vi "LUT_selector.vi"(2 "LUT 2":T1(ring)=enum."cold/hot (1/2)", 3 "LUT1":T1(ring)=enum."cold/hot (1/2)") -> (0 "Palette 2":cluster{u8, u8, u8}[](array[cluster]), 1 "Palette1":cluster{u8, u8, u8}[](array[cluster]))   [LabVIEW 2013]
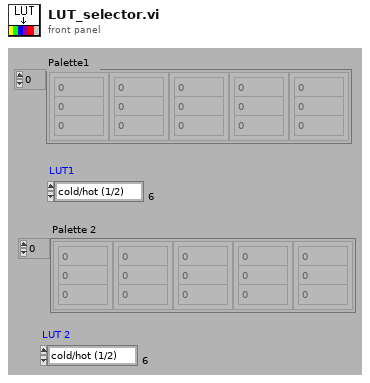
[diagram p1: front panel]
types:
  T1 = enum16{"grey-progress", "gray", "gray + high", "gray + bounds", "gradient", "temperature", "cold/hot (1/2)", "cold/hot (1/4)", "odd/even"}
  T2 = enum32{"Gray", "Binary", "Gradient", "Rainbow", "Temperature"}
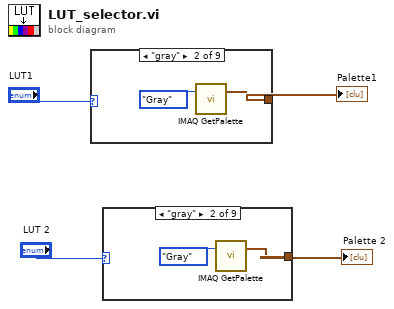
[diagram p0: block diagram]
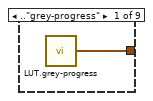
[diagram p2: hidden frame]
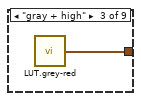
[diagram p3: hidden frame]
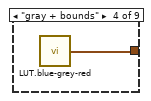
[diagram p4: hidden frame]
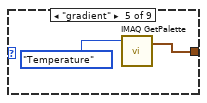
[diagram p5: hidden frame]
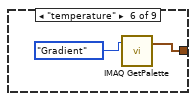
[diagram p6: hidden frame]
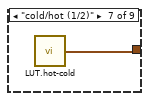
[diagram p7: hidden frame]
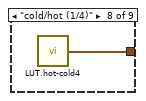
[diagram p8: hidden frame]
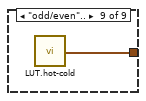
[diagram p9: hidden frame]
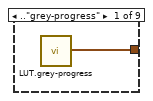
[diagram p10: hidden frame]
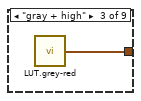
[diagram p11: hidden frame]
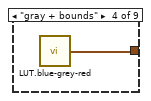
[diagram p12: hidden frame]
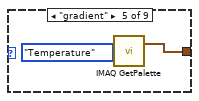
[diagram p13: hidden frame]
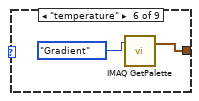
[diagram p14: hidden frame]
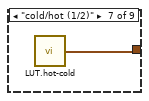
[diagram p15: hidden frame]
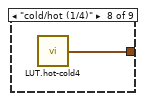
[diagram p16: hidden frame]
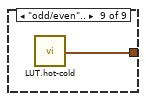
[diagram p17: hidden frame]
diagram:
  n1 = case shown="\"gray\"" "LUT1" {
    tunnel: [w5 w6 w8 w9 w10 w12 w14 w15 w16] -> w4
    frame .."grey-progress" {
      n2 = call "LUT.grey-progress.vi"() -> ("grey-progress"=w5:cluster{u8, u8, u8}[])
    }
    frame "gray" {
      n3 = call "IMAQ GetPalette"("Palette Number (gray)"=T2."Gray") -> ("Color Palette"=w6:cluster{"Red":u8, "Green":u8, "Blue":u8}[])  [unwired: 1 in, 4 out]
    }
    frame "gray + high" {
      n4 = call "LUT.grey-red.vi"() -> ("grey-red Palette"=w8:cluster{u8, u8, u8}[])
    }
    frame "gray + bounds" {
      n5 = call "LUT.blue-grey-red.vi"() -> ("Blue-grey-red Palette"=w9:cluster{u8, u8, u8}[])
    }
    frame "gradient" {
      n6 = call "IMAQ GetPalette"("Palette Number (gray)"=T2."Temperature") -> ("Color Palette"=w10:cluster{"Red":u8, "Green":u8, "Blue":u8}[])  [unwired: 1 in, 4 out]
    }
    frame "temperature" {
      n7 = call "IMAQ GetPalette"("Palette Number (gray)"=T2."Gradient") -> ("Color Palette"=w12:cluster{"Red":u8, "Green":u8, "Blue":u8}[])  [unwired: 1 in, 4 out]
    }
    frame "cold/hot (1/2)" {
      n8 = call "LUT.hot-cold.vi"() -> ("Palette"=w14:cluster{u8, u8, u8}[])
    }
    frame "cold/hot (1/4)" {
      n9 = call "LUT.hot-cold4.vi"() -> ("Palette"=w15:cluster{u8, u8, u8}[])
    }
    frame "odd/even".. {
      n10 = call "LUT.hot-cold.vi"() -> ("Palette"=w16:cluster{u8, u8, u8}[])
    }
  }
  "Palette1" <- w4
  n11 = case shown="\"gray\"" "LUT 2" {
    tunnel: [w17 w18 w20 w21 w23 w24 w26 w27 w28] -> w3
    frame .."grey-progress" {
      n12 = call "LUT.grey-progress.vi"() -> ("grey-progress"=w17:cluster{u8, u8, u8}[])
    }
    frame "gray" {
      n13 = call "IMAQ GetPalette"("Palette Number (gray)"=T2."Gray") -> ("Color Palette"=w18:cluster{"Red":u8, "Green":u8, "Blue":u8}[])  [unwired: 1 in, 4 out]
    }
    frame "gray + high" {
      n14 = call "LUT.grey-red.vi"() -> ("grey-red Palette"=w20:cluster{u8, u8, u8}[])
    }
    frame "gray + bounds" {
      n15 = call "LUT.blue-grey-red.vi"() -> ("Blue-grey-red Palette"=w21:cluster{u8, u8, u8}[])
    }
    frame "gradient" {
      n16 = call "IMAQ GetPalette"("Palette Number (gray)"=T2."Temperature") -> ("Color Palette"=w23:cluster{"Red":u8, "Green":u8, "Blue":u8}[])  [unwired: 1 in, 4 out]
    }
    frame "temperature" {
      n17 = call "IMAQ GetPalette"("Palette Number (gray)"=T2."Gradient") -> ("Color Palette"=w24:cluster{"Red":u8, "Green":u8, "Blue":u8}[])  [unwired: 1 in, 4 out]
    }
    frame "cold/hot (1/2)" {
      n18 = call "LUT.hot-cold.vi"() -> ("Palette"=w26:cluster{u8, u8, u8}[])
    }
    frame "cold/hot (1/4)" {
      n19 = call "LUT.hot-cold4.vi"() -> ("Palette"=w27:cluster{u8, u8, u8}[])
    }
    frame "odd/even".. {
      n20 = call "LUT.hot-cold.vi"() -> ("Palette"=w28:cluster{u8, u8, u8}[])
    }
  }
  "Palette 2" <- w3
